vi "CoreCorelationCalculate.vi"(11 "Cluster":T1) -> ()   [LabVIEW 2024]
uses:
  Core/#CoreQueues.ctl
  vision/#QueueEnum.ctl
  <vilib>/vision/Image Controls.llb/IMAQ Image.ctl
  GUI/#GuiQueueElement.ctl
  GUI/#GuiEnum.ctl
  #CorrelationQueueElement.ctl
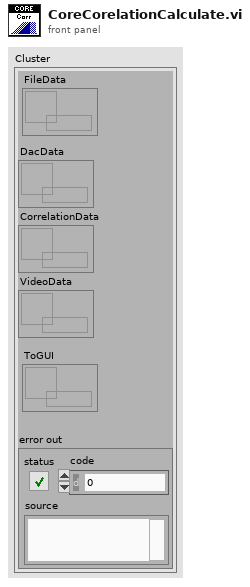
[diagram p1: front panel]
types:
  T1 = typedef "#CoreQueues.ctl" = cluster{"DacData":refnum<queue>, "CorrelationData":refnum<queue>, "VideoData":refnum<queue>, "error out":errorcluster, "ToGUI":refnum<queue>, "FileData":refnum<queue>}
  T2 = cluster{"Antennas":cluster{"Data":dbl[], "t0":timestamp}, "Video":cluster{"Data":dbl[], "t0":timestamp}}
  T3 = typedef "#GuiEnum.ctl" = enum16{"AudioData", "VisionDistances", "DacDistances", "CorrelationDistances", "Video", "DacAquisition", "FPS"}
  T4 = typedef "#GuiQueueElement.ctl" = cluster{"Enum":T3, "Variant":variant}
  T5 = typedef "#QueueEnum.ctl" = enum16{"Ant", "Video"}
  T6 = cluster{"Antennas":cluster{"Data":dbl[], "t0":timestamp}, "Video":cluster{"Data":dbl[], "t0":timestamp}}[]
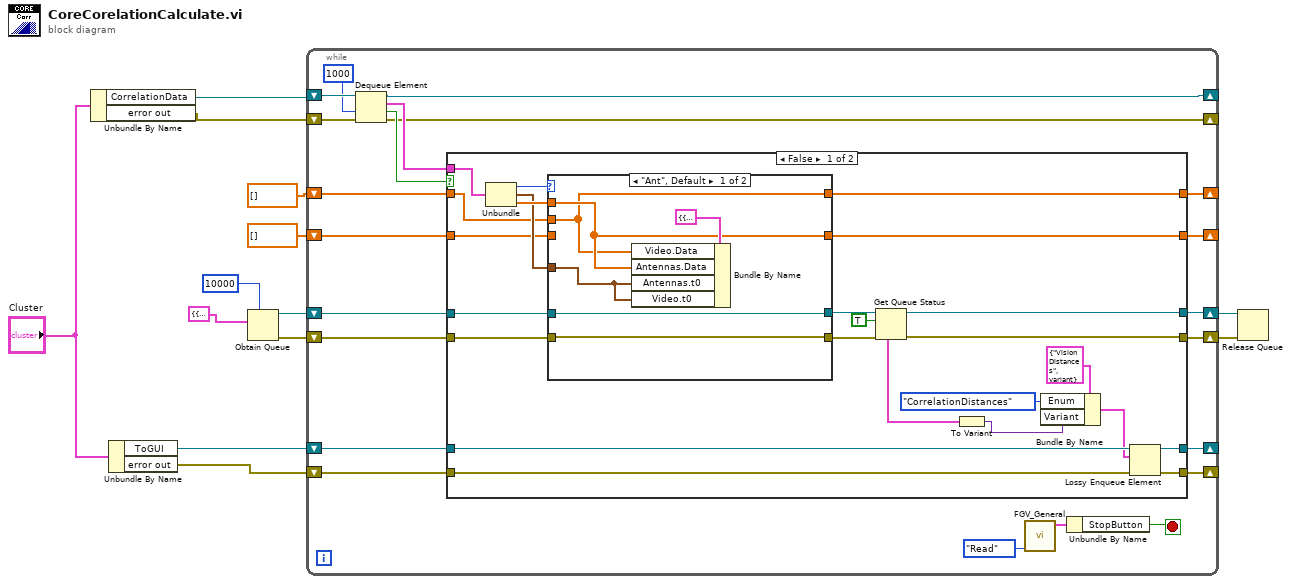
[diagram p0: block diagram]
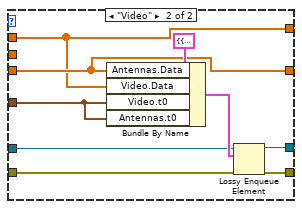
[diagram p2: hidden frame]
diagram:
  n1 = Unbundle By Name("Cluster") -> ("CorrelationData"=w10:refnum<queue>, "error out"=w11:errorcluster)
  n2 = Unbundle By Name("Cluster") -> ("ToGUI"=w12:refnum<queue>, "error out"=w13:errorcluster)
  n3 = Obtain Queue(max queue size (-1, unlimited)=10000, element data type=T2 {"Antennas"={"Data"=[], "t0"=timestamp(0 s since 1904-01-01)}, "Video"={"Data"=[], "t0"=timestamp(0 s since 1904-01-01)}}) -> (queue out=w4:refnum<queue>, error out=w5:errorcluster)  [unwired: 3 in, 1 out]
  n4 = while {
    shift-right: [w25] -> _
    shift-left: w11 -> [w34]
    shift-right: [w26] -> _
    shift-left: w10 -> [w35]
    shift-right: [w28] -> w9
    shift-left: w5 -> [w29]
    shift-right: [w27] -> w8
    shift-left: w4 -> [w30]
    shift-right: [w18] -> _
    shift-left: w12 -> [w21]
    shift-right: [w19] -> _
    shift-left: w13 -> [w20]
    shift-right: [w17] -> _
    shift-left: dbl[] [] -> [w16]
    shift-right: [w15] -> _
    shift-left: dbl[] [] -> [w14]
    stop <- w22 stop-if-true
    n5 = Dequeue Element(queue=w35, timeout in ms (-1)=1000, error in (no error)=w34) -> (queue out=w26:refnum<queue>, element=w31:cluster{"Enum":T5, "t0":timestamp, dbl[]}, timed out?=w32:bool, error out=w25:errorcluster)
    n6 = case shown="False" w32 {
      tunnel: w31 -> [w40 _]
      tunnel: w30 -> [w59 w80]
      tunnel: w29 -> [w58 w79]
      tunnel: [w38 w79] -> w28
      tunnel: [w39 w80] -> w27
      tunnel: w21 -> [w51 w78]
      tunnel: w20 -> [w50 w77]
      tunnel: [w49 w77] -> w19
      tunnel: [w48 w78] -> w18
      tunnel: [w37 w76] -> w17
      tunnel: w16 -> [w42 w76]
      tunnel: [w36 w75] -> w15
      tunnel: w14 -> [w41 w75]
      frame False {
        n7 = Unbundle(w40) -> ("Enum"=w54:T5, "t0"=w52:timestamp, w53:dbl[])
        n8 = case shown="\"Ant\", Default" w54 {
          tunnel: w59 -> [w61 w69]
          tunnel: w58 -> [w60 w74]
          tunnel: w53 -> [w64 w66]
          tunnel: [w60 w73] -> w56
          tunnel: [w61 w72] -> w57
          tunnel: w52 -> [w63 w68]
          tunnel: [w64 w67] -> w37
          tunnel: w42 -> [_ w67]
          tunnel: [w62 w66] -> w36
          tunnel: w41 -> [w62 _]
          frame "Ant", Default {
            n9 = Bundle By Name(cluster=T2 {"Antennas"={"Data"=[], "t0"=timestamp(0 s since 1904-01-01)}, "Video"={"Data"=[], "t0"=timestamp(0 s since 1904-01-01)}}, "Video.Data"=w62, "Antennas.Data"=w64, "Antennas.t0"=w63, "Video.t0"=w63) -> ()  [unwired: 1 out]
          }
          frame "Video" {
            n10 = Bundle By Name(cluster=T2 {"Antennas"={"Data"=[], "t0"=timestamp(0 s since 1904-01-01)}, "Video"={"Data"=[], "t0"=timestamp(0 s since 1904-01-01)}}, "Antennas.Data"=w67, "Video.Data"=w66, "Video.t0"=w68, "Antennas.t0"=w68) -> (w71:T2)
            n11 = Lossy Enqueue Element(queue=w69, element=w71, error in (no error)=w74) -> (queue out=w72:refnum<queue>, error out=w73:errorcluster)  [unwired: 2 out]
          }
        }
        n12 = Get Queue Status(queue=w57, return elements? (F)=TRUE, error in (no error)=w56) -> (queue out=w39:refnum<queue>, error out=w38:errorcluster, elements=w43:T6)  [unwired: 5 out]
        n13 = To Variant(anything=w43) -> (Variant=w44:variant)
        n14 = Bundle By Name(cluster=T4 {"Enum"=enum."VisionDistances", "Variant"=variant} ("element"), "Enum"=#GuiEnum."CorrelationDistances", "Variant"=w44) -> (w45:T4)
        n15 = Lossy Enqueue Element(queue=w51, element=w45, error in (no error)=w50) -> (queue out=w48:refnum<queue>, error out=w49:errorcluster)  [unwired: 2 out]
      }
      frame True {
      }
    }
    n16 = call "FGV_General.vi"("Type"=enum16{"Read", "Write"}."Read") -> ("GeneralIndicator"=w23:cluster{"StartButton":bool, "StopButton":bool})  [unwired: 10 in]
    n17 = Unbundle By Name(w23) -> ("StopButton"=w22:bool)
  }
  n18 = Release Queue(queue=w8, error in (no error)=w9) -> ()  [unwired: 1 in, 3 out]
